vi "Build Table.vi"(7 "Instrument":string, 8 "error in":errorcluster, 9 "variables":string[](array[string]), 11 "stats in":refnum<class "stats.lvclass">) -> (0 "error out":errorcluster, 3 "stats out":refnum<class "stats.lvclass">)   [LabVIEW 2012, in "stats.lvclass"]
uses:
  stats.lvclass
  stats.lvclass/stats.ctl
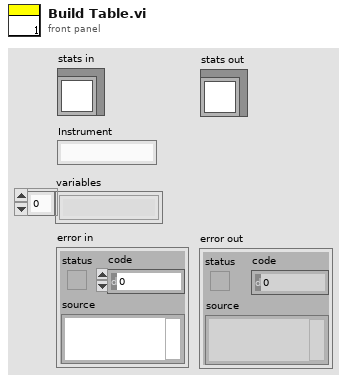
[diagram p1: front panel]
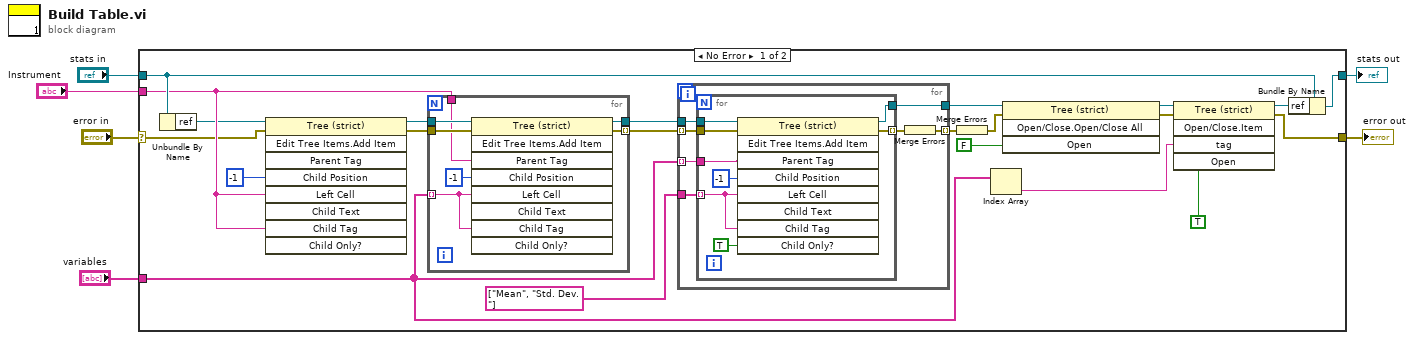
[diagram p0: block diagram]
diagram:
  n1 = case shown="No Error" "error in" {
    selector: "error in" -> [w8 w52]
    tunnel: [w13 w52] -> w5
    tunnel: [w23 w51] -> w3
    tunnel: "stats in" -> [w24 w51]
    tunnel: "variables" -> [w19 _]
    tunnel: "Instrument" -> [w9 _]
    frame No Error {
      n2 = Unbundle By Name(w24) -> ("ref"=w7:refnum<vi>)
      n3 = invoke class="Tree (strict)" method="Edit Tree Items.Add Item"(reference=w7, error in=w8, "Child Position"=-1, "Left Cell"=w9, "Child Tag"=w9) -> (reference out=w12:refnum<vi>, error out=w11:errorcluster)  [unwired: 4 in, 7 out]
      n4 = for {
        tunnel: w12 -> [w50]
        tunnel: w19 -> [w48] mode=indexing
        tunnel: [w47] -> w28
        tunnel: w11 -> [w46]
        tunnel: [w45] -> w27 mode=indexing
        tunnel: w9 -> [w44]
        n5 = invoke class="Tree (strict)" method="Edit Tree Items.Add Item"(reference=w50, error in=w46, "Parent Tag"=w44, "Child Position"=-1, "Left Cell"=w48, "Child Tag"=w48) -> (reference out=w47:refnum<vi>, error out=w45:errorcluster)  [unwired: 3 in, 7 out]
      }
      n6 = for {
        tunnel: w19 -> [w35] mode=indexing
        tunnel: w28 -> [w34]
        tunnel: w27 -> [w33] mode=indexing
        tunnel: string[] ["Mean", "Std. Dev."] ("variables") -> [w32]
        tunnel: [w30] -> w25 mode=indexing
        tunnel: [w29] -> w22
        n7 = for {
          tunnel: w35 -> [w42]
          tunnel: w34 -> [w41]
          tunnel: w33 -> [w40]
          tunnel: w32 -> [w39] mode=indexing
          tunnel: [w38] -> w31 mode=indexing
          tunnel: [w37] -> w29
          n8 = invoke class="Tree (strict)" method="Edit Tree Items.Add Item"(reference=w41, error in=w40, "Parent Tag"=w42, "Child Position"=-1, "Left Cell"=w39, "Child Tag"=w39, "Child Only?"=TRUE) -> (reference out=w37:refnum<vi>, error out=w38:errorcluster)  [unwired: 2 in, 7 out]
        }
        n9 = Merge Errors(w31) -> (w30:errorcluster)
      }
      n10 = Merge Errors(w25) -> (w20:errorcluster)
      n11 = Index Array(array=w19) -> (element=w18:string)  [unwired: 1 in]
      n12 = invoke class="Tree (strict)" method="Open/Close.Open/Close All"(reference=w22, error in=w20, "Open"=FALSE ("Open?")) -> (reference out=w16:refnum<vi>, error out=w15:errorcluster)  [unwired: 1 in, 2 out]
      n13 = invoke class="Tree (strict)" method="Open/Close.Item"(reference=w16, error in=w15, "tag"=w18, "Open"=TRUE ("Open?")) -> (reference out=w14:refnum<vi>, error out=w13:errorcluster)  [unwired: 1 in, 3 out]
      n14 = Bundle By Name(cluster=w24, "ref"=w14) -> (w23:refnum<class "stats.lvclass">)
    }
    frame Error {
    }
  }
  "error out" <- w5
  "stats out" <- w3
